vi "CC Read Channel buffered.vi"(7 "Current File":path, 8 "error in (no error)":errorcluster, 10 "channel":string, 11 "group":string) -> (0 "error out":errorcluster, 2 "Units":string, 3 "Data":cluster{"timestamps":timestamp[], "data":dbl[]})   [LabVIEW 2024]
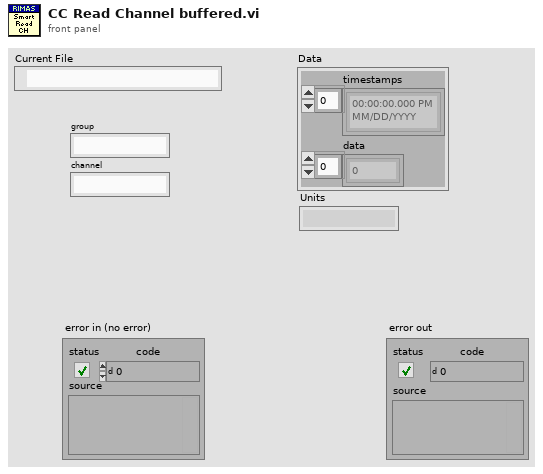
[diagram p1: front panel]
types:
  T1 = cluster{"Offset":i64, "Units":string, "data":dbl[], "timestamps":timestamp[]}
  T2 = enum16{"open", "open or create", "create or replace", "create", "open (read-only)"}
  T3 = map{string, cluster{"Offset":i64, "Units":string, "data":dbl[], "timestamps":timestamp[]}}
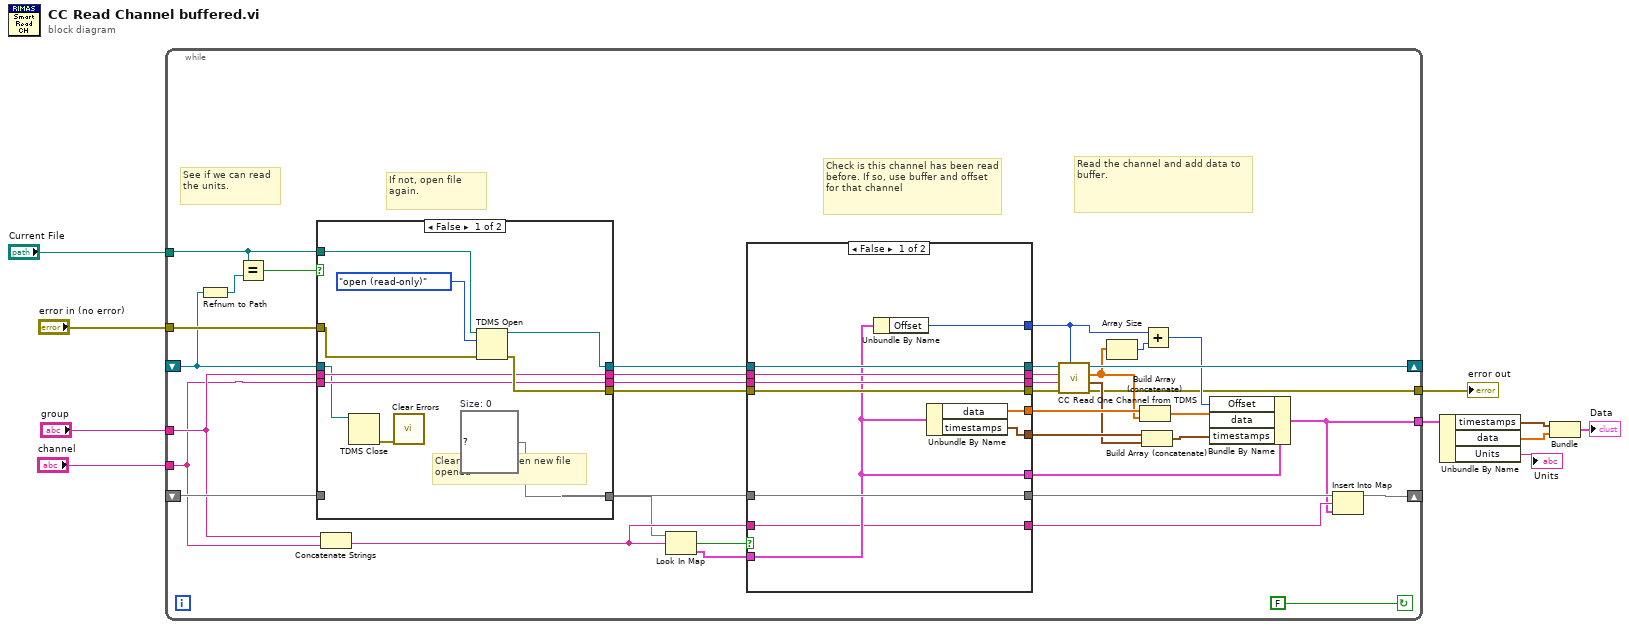
[diagram p0: block diagram]
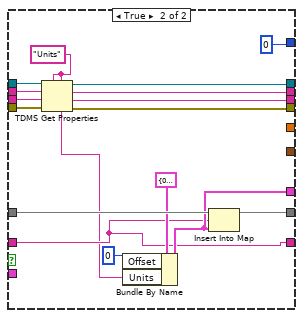
[diagram p2: hidden frame]
diagram:
  n1 = while {
    shift-right: [w47] -> _
    shift-left: _ -> [w14]
    tunnel: "channel" -> [w12]
    tunnel: "group" -> [w13]
    shift-right: [w23] -> _
    shift-left: _ -> [w20]
    tunnel: [w19] -> w8
    tunnel: [w18] -> w7
    tunnel: "error in (no error)" -> [w17]
    tunnel: "Current File" -> [w11]
    stop <- FALSE continue-if-true
    # "Read the channel and add data to buffer."
    # "Check is this channel has been read before. If so, use buffer and offset for that channel"
    # "If not, open file again."
    # "See if we can read the units."
    n2 = Refnum to Path(1:w14) -> (0:w16:path)
    n3 = Equal?(x=w11, y=w16) -> (x = y?=w15:bool)
    n4 = case shown="False" w15 {
      tunnel: w14 -> [w76 w89]
      tunnel: [w79 w89] -> w45
      tunnel: w13 -> [w80 w88]
      tunnel: w12 -> [w81 w87]
      tunnel: [w82 w85] -> w44
      tunnel: [w80 w88] -> w41
      tunnel: [w81 w87] -> w39
      tunnel: [w83 w86] -> w21
      tunnel: w20 -> [_ w86]
      tunnel: w17 -> [w78 w85]
      tunnel: w11 -> [w77 _]
      frame False {
        w83 = T3 {}  # Size: 0
        # "Clear the map when new file\nopened"
        n5 = TDMS Close(11:w76) -> (0:w75:errorcluster)  [unwired: 1 in, 1 out]
        n6 = call <vilib>:"Clear Errors.vi"("error in (no error)"=w75) -> ()  [unwired: 5 in, 2 out]
        n7 = TDMS Open(8:w78, 10:T2."open (read-only)" ("operation (0:open)"), 11:w77) -> (0:w82:errorcluster, 3:w79:refnum<k34>)  [unwired: 4 in]
      }
      frame True {
      }
    }
    n8 = Concatenate Strings(w13, w12) -> (w37:string)
    n9 = Look In Map(map=w21, key=w37) -> (key not found?=w46:bool, value=w43:T1)  [unwired: 1 in]
    n10 = case shown="False" w46 {
      tunnel: w45 -> [w56 w67]
      tunnel: w44 -> [w52 w63]
      tunnel: w43 -> [w49 _]
      tunnel: [w57 i64 0 ("Offset")] -> w26
      tunnel: [w56 w66] -> w42
      tunnel: w41 -> [w55 w65]
      tunnel: [w55 w60] -> w40
      tunnel: w39 -> [w54 w64]
      tunnel: [w54 w59] -> w38
      tunnel: w21 -> [w53 w74]
      tunnel: w37 -> [w48 w68]
      tunnel: [w53 w72] -> w24
      tunnel: [w52 w58] -> w35
      tunnel: [w51 _] -> w34
      tunnel: [w50 _] -> w33
      tunnel: [w49 w69] -> w31
      tunnel: [w48 w68] -> w22
      frame False {
        n11 = Unbundle By Name(w49) -> ("Offset"=w57:i64)
        n12 = Unbundle By Name(w49) -> ("data"=w51:dbl[], "timestamps"=w50:timestamp[])
      }
      frame True {
        w62 = "Units" ("property name")
        n13 = TDMS Get Properties(5:w62, 7:w62, 8:w63, 9:w64, 10:w65, 11:w67) -> (0:w58:errorcluster, 1:w59:string, 2:w60:string, 3:w66:refnum<k34>, 4:w61:string)  [unwired: 1 out]
        n14 = Bundle By Name(cluster=T1 {"Offset"=0, "Units"="", "data"=[], "timestamps"=[]}, "Offset"=0, "Units"=w61) -> (w69:T1)
        n15 = Insert Into Map(map in=w74, key=w68, value=w69) -> (map out=w72:T3)  [unwired: 2 out]
      }
    }
    n16 = call "CC Read One Channel from TDMS.vi"("offset (0)"=w26, "error in (no error)"=w35, "channel"=w38, "group"=w40, "tdms file in"=w42) -> ("error out"=w19:errorcluster, "timestamps"=w32:timestamp[], "data"=w28:dbl[], "tdms file out"=w47:refnum<k34>)  [unwired: 2 in, 1 out]
    n17 = Array Size(array=w28) -> (size(s)=w27:i32)
    n18 = Build Array (concatenate)(w34, w28) -> (w29:dbl[])
    n19 = Build Array (concatenate)(w33, w32) -> (w30:timestamp[])
    n20 = Add(x=w26, y=w27) -> (x+y=w25:i64)
    n21 = Bundle By Name(cluster=w31, "Offset"=w25, "data"=w29, "timestamps"=w30) -> (w18:T1)
    n22 = Insert Into Map(map in=w24, key=w22, value=w18) -> (map out=w23:T3)  [unwired: 2 out]
  }
  "error out" <- w8
  n23 = Unbundle By Name(w7) -> ("timestamps"=w6:timestamp[], "data"=w5:dbl[], "Units"=→"Units":string)
  n24 = Bundle("timestamps"=w6, "data"=w5) -> (→"Data":cluster{"timestamps":timestamp[], "data":dbl[]})  [unwired: 1 in]
